vi "SeqMgr.Populate Seq Step Vars.vi"(8 "error in":errorcluster, 10 "Seq Step In":string[](array[string]), 11 "Variable Values":variant) -> (0 "error out":errorcluster, 2 "Seq Step Out":string[](array[string]))   [LabVIEW 2024, in "EQMF.lvlib" / "SeqMgr.lvlib"]
uses:
  SeqMgr.lvlib
  <vilib>/Utility/error.llb/Trim Whitespace One-Sided.vi
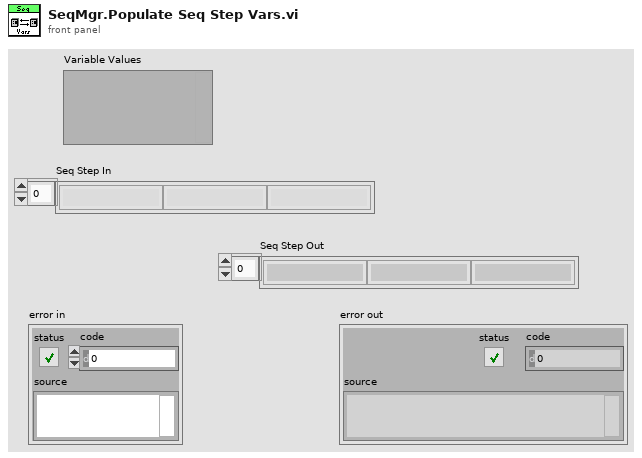
[diagram p1: front panel]
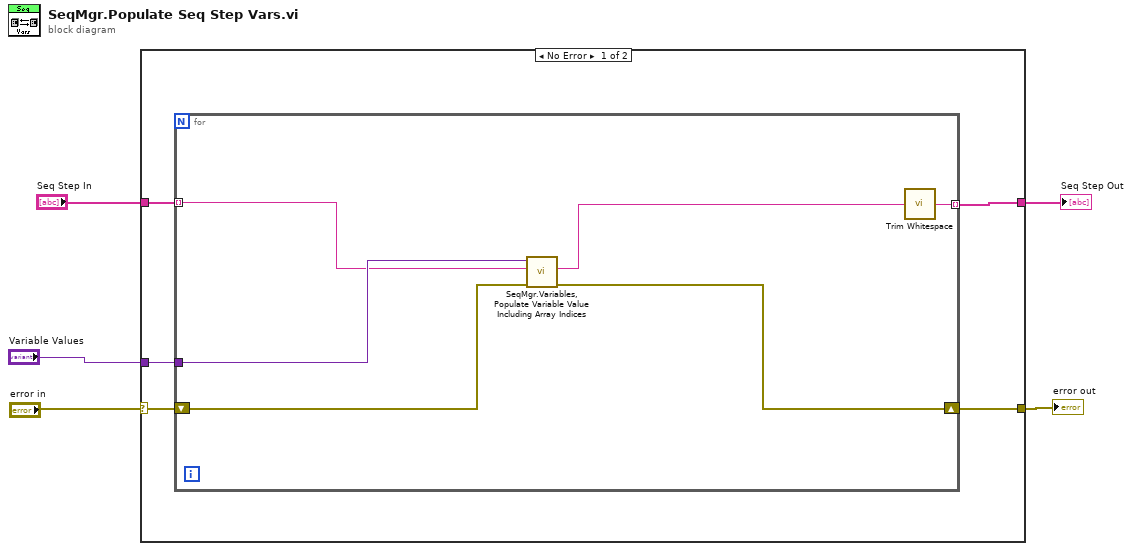
[diagram p0: block diagram]
diagram:
  n1 = case shown="No Error" "error in" {
    selector: "error in" -> [w6 w18]
    tunnel: [w10 w17] -> w1
    tunnel: [w7 w18] -> w4
    tunnel: "Variable Values" -> [w9 _]
    tunnel: "Seq Step In" -> [w8 w17]
    frame No Error {
      n2 = for {
        tunnel: [w16] -> w10 mode=indexing
        tunnel: w9 -> [w15]
        tunnel: w8 -> [w14] mode=indexing
        shift-right: [w12] -> w7
        shift-left: w6 -> [w11]
        n3 = call "SeqMgr.Variables, Populate Variable Value Including Array Indices.vi"("error in"=w11, "String"=w14, "Variables"=w15) -> ("error out"=w12:errorcluster, "String Out"=w13:string)  [unwired: 6 in, 1 out]
        n4 = call <vilib>:"Trim Whitespace.vi"("string"=w13) -> ("trimmed string"=w16:string)  [unwired: 1 in]
      }
    }
    frame Error {
    }
  }
  "error out" <- w4
  "Seq Step Out" <- w1
